vi "calcStuff.vi"(9 "VRefn":dbl, 10 "VRefp":dbl, 11 "Data":i32[](array[numeric])) -> (2 "stepSize(V)":dbl format="%#.20f", 3 "nOfSteps":i32)   [LabVIEW 2014]
panel:
  in  "c":i32 format="%032b"
  out "i":i32
  out "outb":u32
  in  "outb2":bool
  in  "outb1":bool
  in  "outb0":bool
  out "a & b":i32
  in  "b":i32 format="%032b"
  in  "a":i32 format="%032b"
  out "x > 0?":bool
  in  "Numeric":i32
  in  "start":i32 format="%032b"
  out "nextVolt":i32 format="%032b"
  out "-stepSize":i32 format="%032b"
  in  "stepSize":i32 format="%032b"
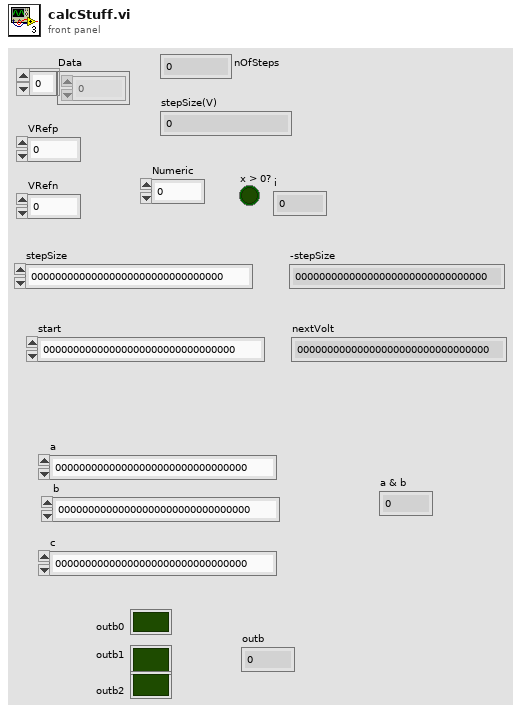
[diagram p1: front panel]
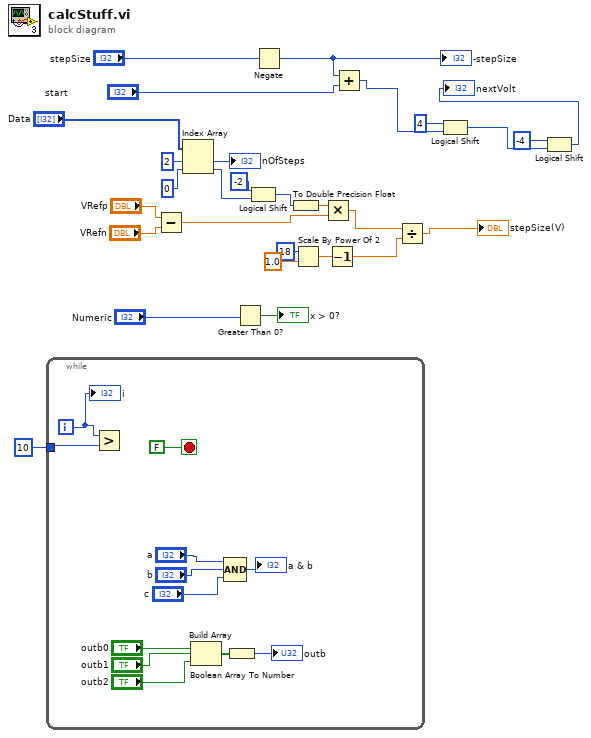
[diagram p0: block diagram]
diagram:
  n1 = while {
    tunnel: 10 -> [w31]
    i -> [w32]
    stop <- FALSE stop-if-true
    n2 = Greater?(x=w32, y=w31) -> ()  [unwired: 1 out]
    n3 = Build Array("outb0", "outb1", "outb2") -> (w37:bool[])
    n4 = Compound Arithmetic op=AND("a", "b", "c") -> (→"a & b":i32)
    n5 = Boolean Array To Number(Boolean array=w37) -> (number=→"outb":u32)
    "i" <- w32
  }
  n6 = Subtract(x="VRefp", y="VRefn") -> (x-y=w19:dbl)
  n7 = Index Array(array="Data", index #1=2 ("index"), index #2=0 ("index")) -> (element #1=→"nOfSteps":i32, element #2=w16:i32)
  n8 = Greater Than 0?(x="Numeric") -> (x > 0?=→"x > 0?":bool)
  n9 = Logical Shift(y=i16 -2, x=w16) -> (x << y=w18:i32)
  n10 = Negate(x="stepSize") -> (-x=w9:i32)
  "-stepSize" <- w9
  n11 = To Double Precision Float(number=w18) -> (double precision float=w20:dbl)
  n12 = Scale By Power Of 2(n=i16 18, x=1.0) -> (x*2^n=w23:dbl)
  n13 = Multiply(x=w20, y=w19) -> (x*y=w24:dbl)
  n14 = Decrement(x=w23) -> (x-1=w25:dbl)
  n15 = Add(x=w9, y="start") -> (x+y=w5:i32)
  n16 = Divide(x=w24, y=w25) -> (x/y=→"stepSize(V)":dbl)
  n17 = Logical Shift(y=i16 4, x=w5) -> (x << y=w6:i32)
  n18 = Logical Shift(y=i16 -4, x=w6) -> (x << y=→"nextVolt":i32)
